vi "4.6.3.vi"() -> ()   [LabVIEW 2017]
panel:
  in  "停止":bool
  out "数值 3":dbl
  in  "数值 2":dbl
  in  "数值":dbl
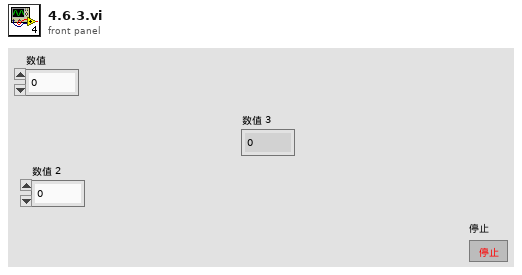
[diagram p1: front panel]
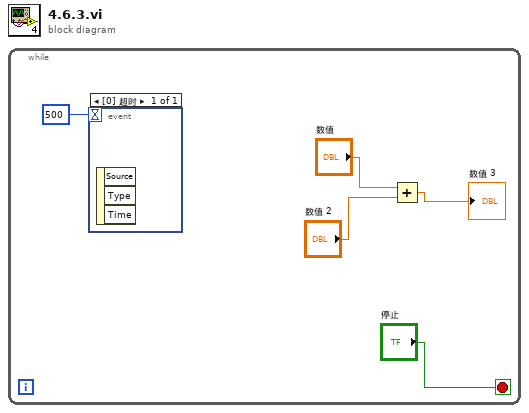
[diagram p0: block diagram]
diagram:
  n1 = while {
    stop <- "停止" stop-if-true
    n2 = event shown="[0] 超时" {
      selector: _ -> [_]
      dyn-events: _ -> [_]
      timeout: 500 -> [_]
      event Timeout {
        n3 = event-data() -> ()  [unwired: 1 in, 3 out]
      }
    }
    n4 = Add(x="数值", y="数值 2") -> (x+y=→"数值 3":dbl)
  }
